vi "waveformdatatype.vi"() -> ()   [LabVIEW 2019]
panel:
  out "size(s)":i32[](array[numeric])
  out "Waveform Graph 3":i32[](graph)
  out "Waveform Chart 2":i32[](graph)
  out "Waveform Graph 2":dbl[][](graph)
  out "x^3":cluster{i32, i32, i32[]}(graph)
  out "Waveform Graph":i32[](graph)
  out "Waveform Chart":dbl(graph)
  in  "stop":bool
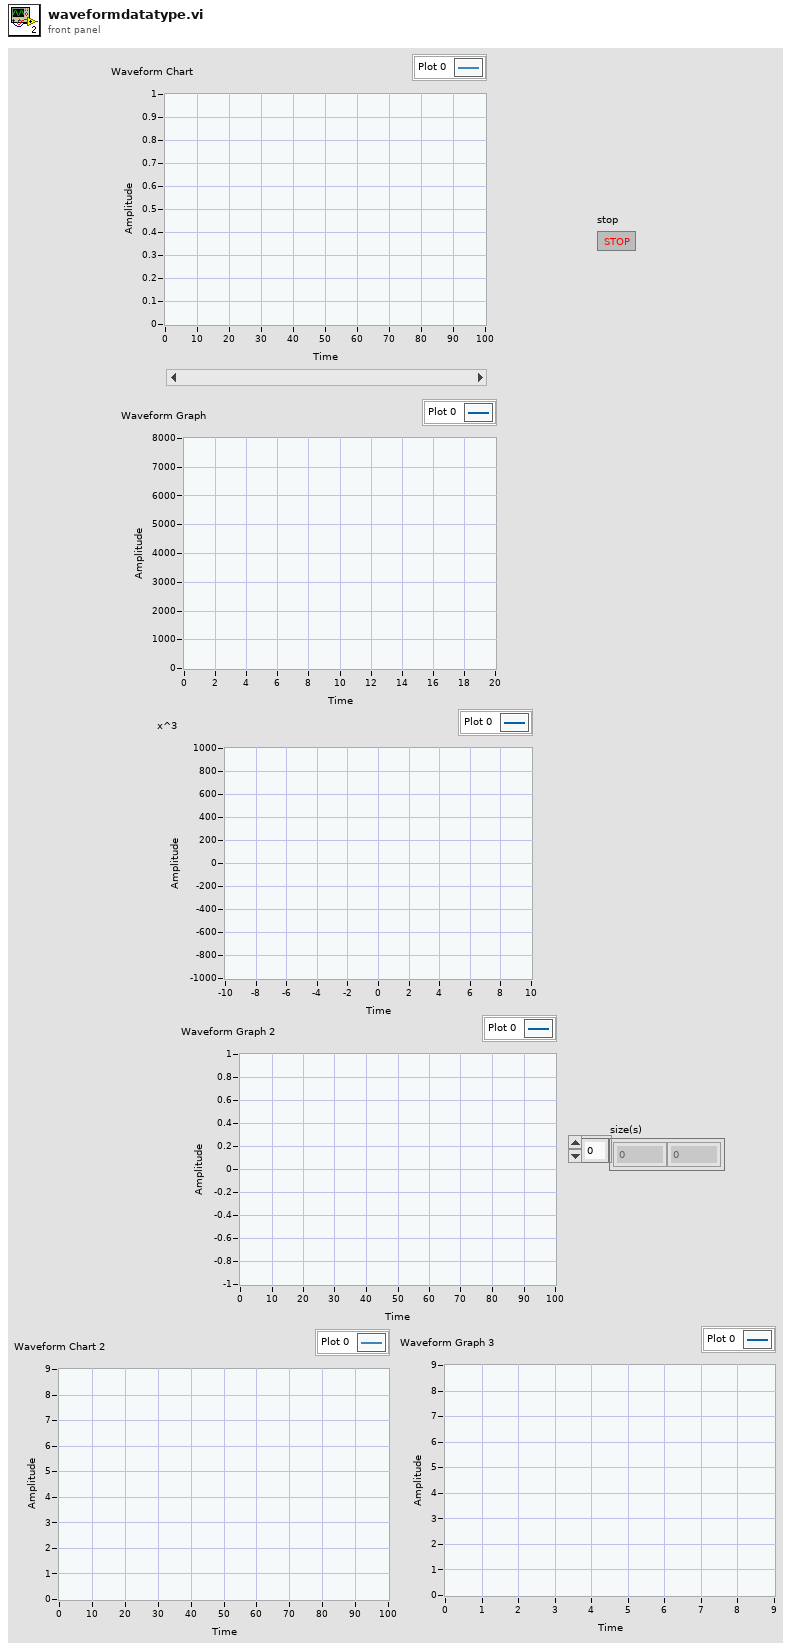
[diagram p1: front panel]
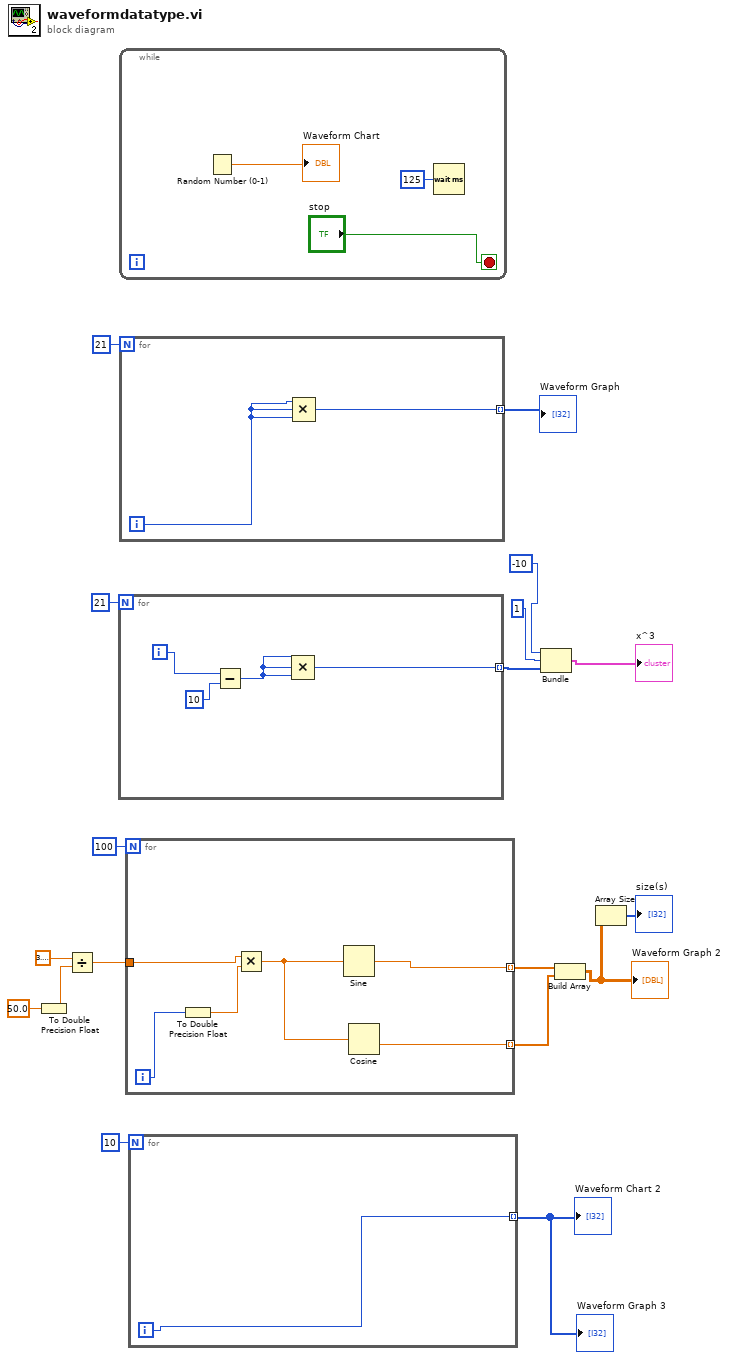
[diagram p0: block diagram]
diagram:
  n1 = To Double Precision Float(number=50.0) -> (double precision float=w9:dbl)
  n2 = Divide(x=3.141592653589793, y=w9) -> (x/y=w7:dbl)
  n3 = for {
    N: 21 -> [_]
    tunnel: [w22] -> w15 mode=indexing
    i -> [w21]
    n4 = Subtract(x=w21, y=10) -> (x-y=w19:i32)
    n5 = Compound Arithmetic op=MULTIPLY(w19, w19, w19) -> (w22:i32)
  }
  n6 = while {
    stop <- "stop" stop-if-true
    n7 = Random Number (0-1)() -> (number: 0 to 1=→"Waveform Chart":dbl)
    n8 = Wait (ms)(milliseconds to wait=u32 125) -> ()  [unwired: 1 out]
  }
  n9 = for {
    N: 21 -> [_]
    tunnel: [w26] -> w17 mode=indexing
    i -> [w27]
    n10 = Compound Arithmetic op=MULTIPLY(w27, w27, w27) -> (w26:i32)
  }
  "Waveform Graph" <- w17
  n11 = for {
    N: 100 -> [_]
    tunnel: w7 -> [w33]
    tunnel: [w29] -> w6 mode=indexing
    tunnel: [w28] -> w5 mode=indexing
    i -> [w31]
    n12 = To Double Precision Float(number=w31) -> (double precision float=w32:dbl)
    n13 = Multiply(x=w33, y=w32) -> (x*y=w30:dbl)
    n14 = Sine(x=w30) -> (sin(x)=w29:dbl)
    n15 = Cosine(x=w30) -> (cos(x)=w28:dbl)
  }
  n16 = for {
    N: 10 -> [_]
    tunnel: [w34] -> w3 mode=indexing
    i -> [w34]
  }
  "Waveform Chart 2" <- w3
  "Waveform Graph 3" <- w3
  n17 = Bundle "Bundle"(-10, 1, w15) -> (→"x^3":cluster{i32, i32, i32[]})  [unwired: 1 in]
  n18 = Build Array(w6, w5) -> (w2:dbl[][])
  "Waveform Graph 2" <- w2
  n19 = Array Size(array=w2) -> (size(s)=→"size(s)":i32[])
